vi "Save MDIF File.vi"(7 "Use Numbers For Types (False)":bool, 8 "error in (no error)":errorcluster, 9 "Comment Line Prefix (REM)":i32(ring) items=["REM", "Exclamation"], 10 "Value Separator (Space)":i32(ring) items=["Space", "Tab", "Two Tabs"], 11 "MDIF reference in":refnum<k24>) -> (0 "error out":errorcluster, 3 "MDIF reference out":refnum<k24>)   [LabVIEW 2023, in "NI_HFNetworkAnalysis.lvlib"]
doc: "Save all MDIF blocks in memory to the referenced MDIF file.\n\n<b>Notes</b>\n- If the reference MDIF file already exists, it is overwritten with the MDIF Blocks in memory.\n- Use <b>Close MDIF File.vi</b> to close reference to the MDIF file."
uses:
  NI_HFNetworkAnalysis.lvlib
  C:/srd-semi-rfcal-software/AuxTools/STSRFFixtureCharactUtility/Source/Code Modules/Fixture/Dependencies/HFNetworkAnalysis/Support Files/NACE.Utils.Data.dll
  Support Files/NACE.Utils.Data.dll
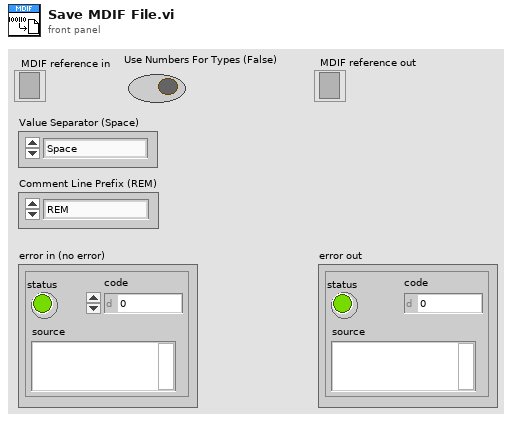
[diagram p1: front panel]
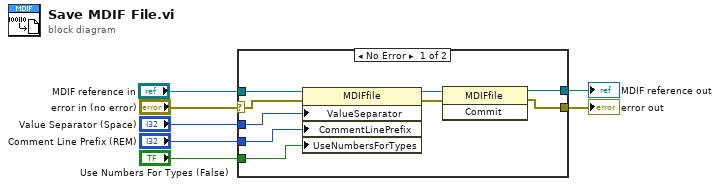
[diagram p0: block diagram]
diagram:
  n1 = case shown="No Error" "error in (no error)" {
    selector: "error in (no error)" -> [w12 w18]
    tunnel: "Value Separator (Space)" -> [w16 _]
    tunnel: "Comment Line Prefix (REM)" -> [w15 _]
    tunnel: "Use Numbers For Types (False)" -> [w14 _]
    tunnel: "MDIF reference in" -> [w13 w17]
    tunnel: [w9 w18] -> w2
    tunnel: [w8 w17] -> w1
    frame No Error {
      n2 = property class="MDIFfile"(reference=w13, error in=w12, "ValueSeparator"=w16, "CommentLinePrefix"=w15, "UseNumbersForTypes"=w14) -> (reference out=w10:refnum<k24>, error out=w11:errorcluster)
      n3 = invoke class="MDIFfile" method="Commit"(reference=w10, error in=w11) -> (reference out=w8:refnum<k24>, error out=w9:errorcluster)  [unwired: 1 in, 1 out]
    }
    frame Error {
    }
  }
  "error out" <- w2
  "MDIF reference out" <- w1
